vi "2 OverrideHandler.vi"() -> ()   [LabVIEW 2011]
uses:
  2 Globals/2 Global.vi
  2 Typedefs/sail setpt.ctl
  2 Typedefs/rudder angle.ctl
  2 Typedefs/setpoints to boat.ctl
panel:
  out "Override Active Rudder":bool
  out "Think Setpoints":cluster{"Rudder Angle":T1, "Sail Position":T2}
  out "Override Active Sail":bool
  out "Override Setpoints":T3
  out "Setpoints to Boat":T3
  # "This is the Override Handler: \nIt checks to see if the manual override has been activated, and sends setpoints to the boat based on that boolean.\n\nTODO: Check to make sure that rudder and sail are always communicated as (0) = rudder and (1) = sail."
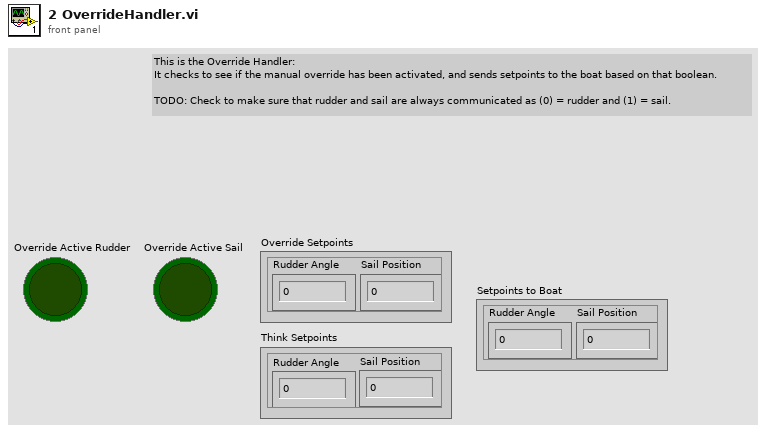
[diagram p1: front panel]
types:
  T1 = typedef "rudder angle.ctl" = dbl
  T2 = typedef "sail setpt.ctl" = dbl
  T3 = typedef "setpoints to boat.ctl" = cluster{"Sail Position":T2, "Rudder Angle":T1}
  T4 = typedef "manual override.ctl" = cluster{"Override Active Rudder":bool, "Setpoints":T3, "Override Active Sail":bool}
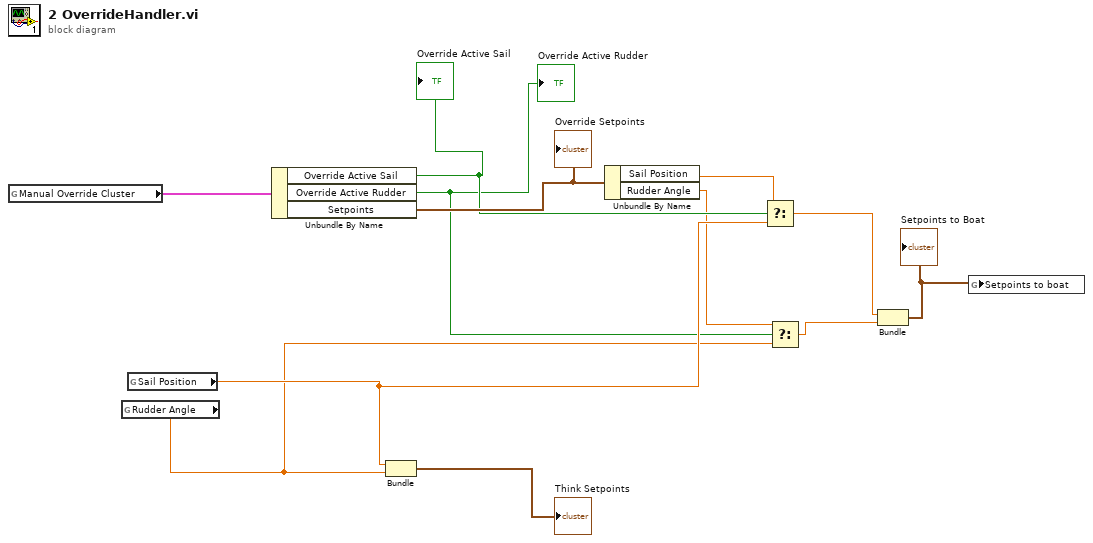
[diagram p0: block diagram]
diagram:
  n1 = global read "2 Global.vi" "Manual Override Cluster"() -> (w12:T4)
  n2 = global read "2 Global.vi" "Rudder Angle"() -> (w4:T1)
  n3 = global read "2 Global.vi" "Sail Position"() -> (w6:T2)
  n4 = Unbundle By Name(w12) -> ("Override Active Sail"=w8:bool, "Override Active Rudder"=w5:bool, "Setpoints"=w10:T3)
  "Override Setpoints" <- w10
  "Override Active Sail" <- w8
  "Override Active Rudder" <- w5
  n5 = Bundle("Sail Position"=w6, "Rudder Angle"=w4) -> (→"Think Setpoints":cluster{"Sail Position":T2, "Rudder Angle":T1})  [unwired: 1 in]
  n6 = Unbundle By Name(w10) -> ("Sail Position"=w7:T2, "Rudder Angle"=w1:T1)
  n7 = Select(t=w7, s=w8, f=w6) -> (s? t:f=w2:T2)
  n8 = Select(t=w1, s=w5, f=w4) -> (s? t:f=w3:T1)
  n9 = Bundle("Sail Position"=w2, "Rudder Angle"=w3) -> (w9:cluster{"Sail Position":T2, "Rudder Angle":T1})  [unwired: 1 in]
  "Setpoints to Boat" <- w9
  n10 = global write "2 Global.vi" "Setpoints to boat"(w9) -> ()
